vi "DB_table_index.vi"(8 "data type":T1, 11 "Thumb":string) -> (3 "column information 2":T2)   [LabVIEW 2016]
uses:
  <vilib>/addons/database/Auxilliary.llb/DB Tools Column Info.ctl
  <vilib>/addons/database/Auxilliary.llb/DB Tools DataTypes.ctl
  <vilib>/addons/database/NI_Database_API.lvlib
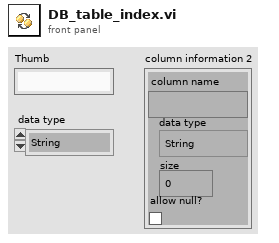
[diagram p1: front panel]
types:
  T1 = typedef "NI_Database_API.lvlib/DB Tools DataTypes.ctl" = enum16{"String", "Long (I32)", "Single (SGL)", "Double (DBL)", "Date/Time", "Binary"}
  T2 = typedef "NI_Database_API.lvlib/DB Tools Column Info.ctl" = cluster{"column name":string, "data type":T1, "size":i32, "allow null?":bool}
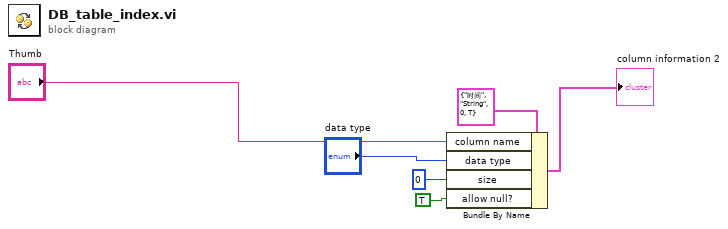
[diagram p0: block diagram]
diagram:
  n1 = Bundle By Name(cluster=T2 {"column name"="时间", "data type"=enum."String", "size"=0, "allow null?"=TRUE} ("column information 2"), "column name"="Thumb", "data type"="data type", "size"=0, "allow null?"=TRUE) -> (→"column information 2":T2)
